vi "Temp_meas_DS18B20.vi"() -> ()   [LabVIEW 2013]
uses:
  <vilib>/rvi/Emulation/niFpgaSctlEmulationGetInTimedLoop.vi
  <vilib>/rvi/Emulation/niFpgaEmulationReportErrorSimple.vi
  <vilib>/rvi/Emulation/niFpgaGetClockAttributes.vi
  <vilib>/rvi/Emulation/niFpgaCriticalErrorInLSC.vi
panel:
  out "error out":errorcluster
  out "Scratchpad Data":u8[](array[numeric])
  out "Temperature (raw)":u16
  out "0 = Device Present / 1=no":bool
  in  "stop":bool
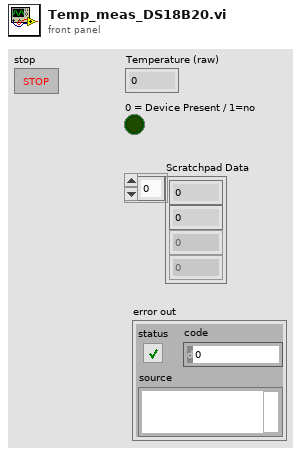
[diagram p1: front panel]
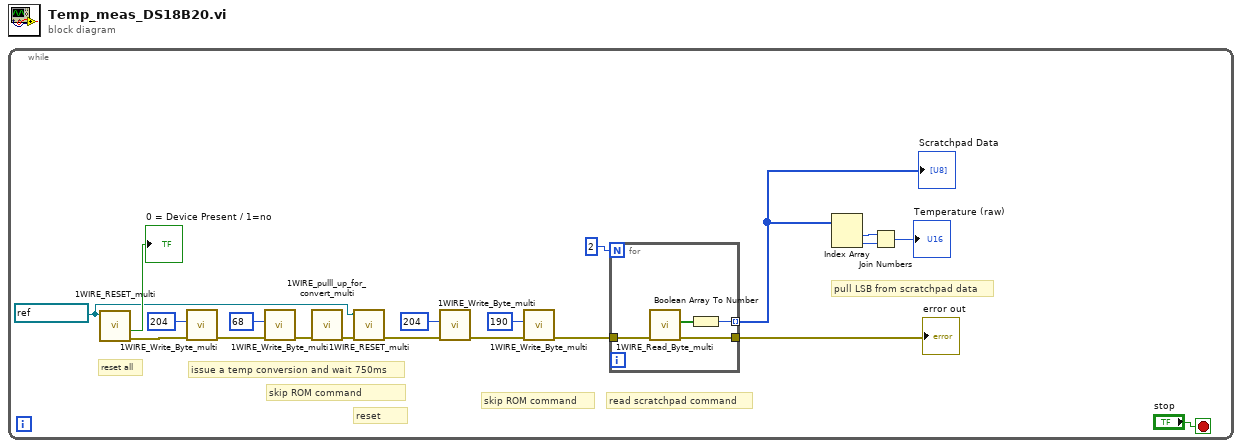
[diagram p0: block diagram]
diagram:
  n1 = while {
    stop <- "stop" stop-if-true
    w1 = refnum<k21> "DS_WIRE" ("FPGA I/O In")
    # "pull LSB from scratchpad data"
    # "read scratchpad command"
    # "skip ROM command"
    # "reset"
    # "issue a temp conversion and wait 750ms"
    # "skip ROM command"
    # "reset all"
    n2 = call "1WIRE_RESET_multi.vi"("FPGA I/O In"=w1) -> ("error out"=w6:errorcluster, "0 = Device Present / 1=no"=→"0 = Device Present / 1=no":bool)  [unwired: 9 in]
    n3 = call "1WIRE_Write_Byte_multi.vi"("error in"=w6, "Tx data"=u8 204 ("Tx data 2")) -> ("error out"=w5:errorcluster)  [unwired: 8 in, 1 out]
    n4 = call "1WIRE_Write_Byte_multi.vi"("error in"=w5, "Tx data"=u8 68 ("Tx data 2")) -> ("error out"=w19:errorcluster)  [unwired: 8 in, 1 out]
    n5 = call "1WIRE_pulll_up_for_convert_multi.vi"("error in"=w19) -> ("error out"=w7:errorcluster)  [unwired: 10 in]
    n6 = call "1WIRE_RESET_multi.vi"("error in"=w7, "FPGA I/O In"=w1) -> ("error out"=w8:errorcluster)  [unwired: 8 in, 1 out]
    n7 = call "1WIRE_Write_Byte_multi.vi"("error in"=w8, "Tx data"=u8 204 ("Tx data 2")) -> ("error out"=w9:errorcluster)  [unwired: 8 in, 1 out]
    n8 = call "1WIRE_Write_Byte_multi.vi"("error in"=w9, "Tx data"=u8 190 ("Tx data 2")) -> ("error out"=w11:errorcluster)  [unwired: 8 in, 1 out]
    n9 = for {
      N: 2 -> [_]
      tunnel: w11 -> [w24]
      tunnel: [w23] -> w2
      tunnel: [w22] -> w14 mode=indexing
      n10 = call "1WIRE_Read_Byte_multi.vi"("error in"=w24) -> ("error out"=w23:errorcluster, "Array"=w21:bool[])  [unwired: 9 in]
      n11 = Boolean Array To Number(Boolean array=w21) -> (number=w22:u8)
    }
    "Scratchpad Data" <- w14
    "error out" <- w2
    n12 = Index Array(array=w14) -> (element #1=w13:u8, element #2=w15:u8)  [unwired: 2 in]
    n13 = Join Numbers(hi=w13, lo=w15) -> ((hi.lo)=→"Temperature (raw)":u16)
  }
